vi "Log Error.vi"(8 "error in (no error)":errorcluster, 9 "error":errorcluster, 10 "state":T1=enum."Start", 11 "Plugin Thread in":refnum<class "Plugin Thread.lvclass">) -> (0 "error out":errorcluster, 3 "Plugin Thread out":refnum<class "Plugin Thread.lvclass">)   [LabVIEW 2017, in "DSF Core.lvlib" / "Plugin Thread.lvclass"]
uses:
  Plugin Thread.lvclass
  C:/Git/DSF/Core/Classes/Thread/Thread.lvclass
  Interface/Plugin/Command.ctl
  <vilib>/NI/Memory Manager/Classes/Pointer/Pointer.lvclass/Pointer.ctl
  Plugin Thread.lvclass/Plugin Thread.ctl
  Interface/Logging/Command Data.ctl
  Interface/Logging/Command.ctl
  Interface/Logging/Parameters.ctl
  Interface/Logging/Plugin State Parameters.ctl
  Pointers/Error/Error Pointer.lvclass
  C:/Program Files (x86)/National Instruments/LabVIEW 2017/vi.lib/NI/Memory Manager/Classes/Pointer/Pointer.lvclass
  Interface/Logging/Send Logging Command.vi
  Interface/Logging/Logging Interface.lvclass
  Thread.lvclass
  <vilib>/NI/Memory Manager/Classes/Pointer/Pointer.lvclass
  Interface/Plugin/Plugin Interface.lvclass
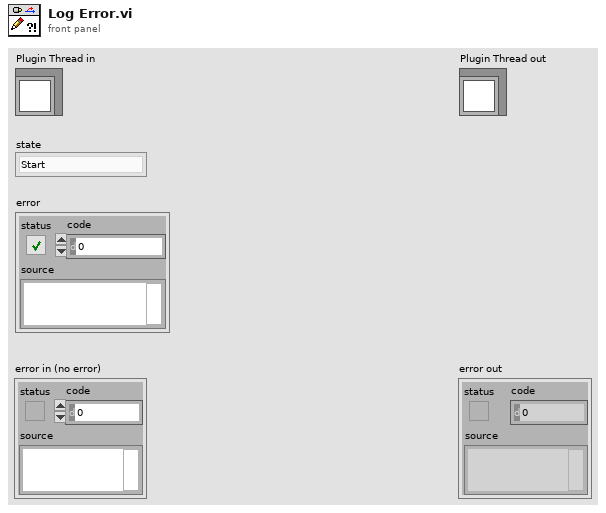
[diagram p1: front panel]
types:
  T1 = typedef "DSF Core.lvlib/Plugin Interface.lvclass/Command.ctl" = enum8{"Idle", "Start", "Set Inline Buffer", "Rx", "Tx", "Shutdown", "Error"}
  T2 = typedef "DSF Core.lvlib/Logging Interface.lvclass/Parameters.ctl" = cluster{"arg1":u64, "arg2":u64}
  T3 = typedef "DSF Core.lvlib/Logging Interface.lvclass/Plugin State Parameters.ctl" = cluster{"state":T1, "Plugin ID":u8, "Thread ID":u8, "unused 0":u8, "unused 1":i32, "error pointer":u64}
  T4 = typedef "DSF Core.lvlib/Logging Interface.lvclass/Command.ctl" = enum8{"Idle", "Start", "Log Framework State", "Log Plugin State", "Log Dispatcher State", "Shutdown"}
  T5 = typedef "DSF Core.lvlib/Logging Interface.lvclass/Command Data.ctl" = cluster{"Command":T4, "Parameters":T2}
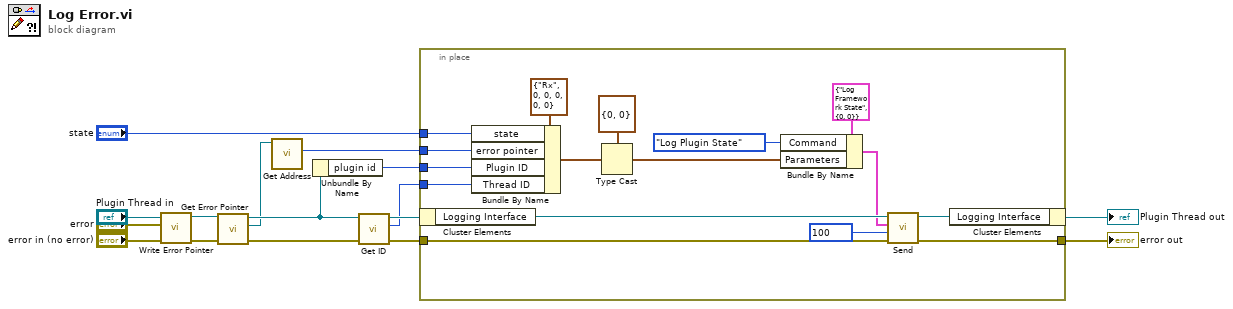
[diagram p0: block diagram]
diagram:
  n1 = call "Write Error Pointer.vi"("error in (no error)"="error in (no error)", "error"="error", "Thread in"="Plugin Thread in") -> ("error out"=w8:errorcluster, "Thread out"=w7:refnum<class "Plugin Thread.lvclass">)  [unwired: 7 in]
  n2 = call "Get Error Pointer.vi"("Thread in"=w7) -> ("error pointer"=w1:refnum<class "Error Pointer.lvclass">, "Thread out"=w4:refnum<class "Plugin Thread.lvclass">)  [unwired: 9 in]
  n3 = call <vilib>:"Get Address.vi"("Pointer in"=w1) -> ("address"=w12:u64)  [unwired: 9 in, 1 out]
  n4 = Unbundle By Name(w4) -> ("plugin id"=w5:i32)
  n5 = call "Get ID.vi"("Thread in"=w4) -> ("ID"=w2:i32, "Thread out"=w3:refnum<class "Plugin Thread.lvclass">)  [unwired: 9 in]
  n6 = in-place {
    in-place-border: [w26] -> w14
    in-place-border: w8 -> [w24]
    in-place-border: "state" -> [w19]
    in-place-border: w12 -> [w17]
    in-place-border: w5 -> [w16]
    in-place-border: w2 -> [w15]
    n7 = in-place-cluster #1(w3) -> ("Logging Interface"=w30:refnum<class "Logging Interface.lvclass">)
    n8 = Bundle By Name(cluster=T3 {"state"=enum."Rx", "Plugin ID"=0, "Thread ID"=0, "unused 0"=0, "unused 1"=0, "error pointer"=0} ("Parameters"), "state"=w19, "error pointer"=w17, "Plugin ID"=w16, "Thread ID"=w15) -> (w22:T3)
    n9 = Type Cast(type=T2 {"arg1"=0, "arg2"=0} ("Parameters"), x=w22) -> (*(type *) &x=w20:T2)
    n10 = Bundle By Name(cluster=T5 {"Command"=enum."Log Framework State", "Parameters"={"arg1"=0, "arg2"=0}} ("command"), "Command"=Command."Log Plugin State", "Parameters"=w20) -> (w27:T5)
    n11 = call-poly "Send.vi"("error in (no error)"=w24, "timeout in ms (0)"=100, "command"=w27, "Logging Interface in"=w30) -> ("error out"=w26:errorcluster, "Logging Interface out"=w25:refnum<class "Logging Interface.lvclass">)  [unwired: 6 in]
    n12 = in-place-cluster #1("Logging Interface"=w25) -> (→"Plugin Thread out":refnum<class "Plugin Thread.lvclass">)
  }
  "error out" <- w14
